vi "solar_voy_def Export (Packets).vi"(10 "HDR_ID_NAME ('HDR_ID')":string="HDR_ID", 11 "PACKETS":T1[](array[typedef]) {"last_time" format="%<%H:%M:%S%3u %m/%d/%y>T"}) -> (2 "Telemetry":string, 3 "Commands":string)   [LabVIEW 2018]
doc: "This exports packets to COSMOS definition strings."
uses:
  solar_voy_def_ctl ITEM TYPE.ctl
  type/solar_type Item Type.ctl
  solar_voy_def_ctl ITEM.ctl
  solar_voy_def_ctl PACKET_ID.ctl
  solar_voy_def_ctl PACKET.ctl
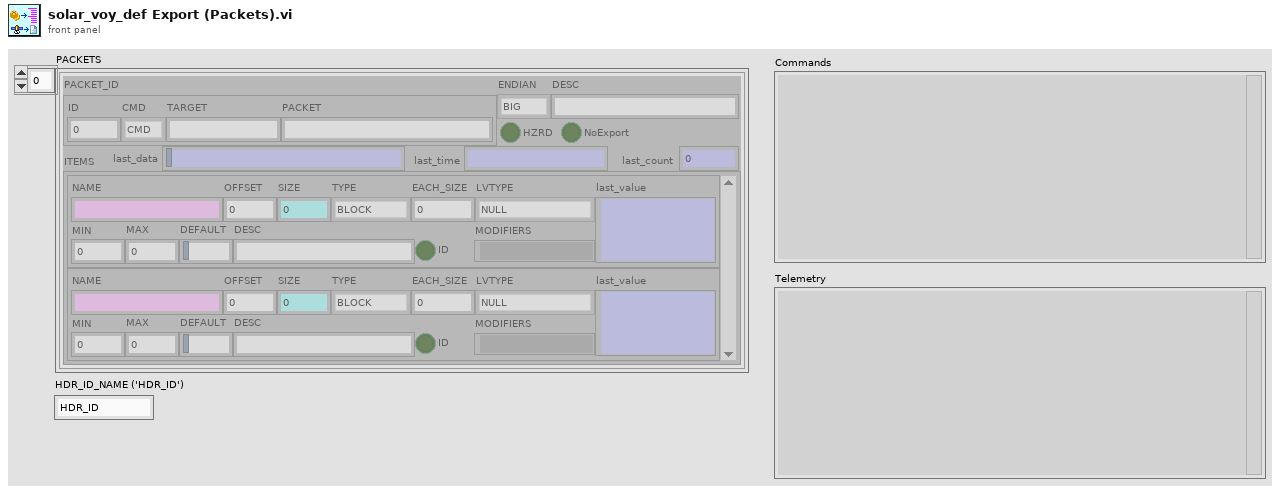
[diagram p1: front panel]
types:
  T1 = typedef "solar_voy_def_ctl PACKET.ctl" = cluster{"PACKET_ID":T2, "ENDIAN":enum8{"BIG", "LITTLE"}, "DESC":string, "HZRD":bool, "ITEMS":T3[], "NoExport":bool, "last_time":timestamp, "last_count":u32, "last_data":string}
  T2 = typedef "solar_voy_def_ctl PACKET_ID.ctl" = cluster{"ID":u16, "CMD":enum8{"CMD", "TLM"}, "TARGET":string, "PACKET":string}
  T3 = typedef "solar_voy_def_ctl ITEM.ctl" = cluster{"NAME":string, "OFFSET":i32, "SIZE":i32, "TYPE":T4, "EACH_SIZE":i32, "LVTYPE":T5, "MIN":dbl, "MAX":dbl, "DEFAULT":string, "DESC":string, "ID":bool, "MODIFIERS":variant, "last_value":variant}
  T4 = typedef "solar_voy_def_ctl ITEM TYPE.ctl" = enum8{"BLOCK", "INT", "UINT", "FLOAT", "STRING"}
  T5 = typedef "solar_type Item Type.ctl" = enum16{"NULL", "UNKNOWN", "CLUSTER", "I8", "I16", "I32", "I64", "U8", "U16", "U32", "U64", "U8_ENUM", "U16_ENUM", "U32_ENUM", "SGL", "DBL", "BOOLEAN", "STRING", "PATH", "VISA", "TAG", "TIME", "I8_1D", "I16_1D", "I32_1D", "I64_1D", "U8_1D", "U16_1D", "U32_1D", "U64_1D", "U8_ENUM_1D", "U16_ENUM_1D", "U32_ENUM_1D", "SGL_1D", "DBL_1D", "BOOLEAN_1D", "STRING_1D", "PATH_1D", "VISA_1D", "TAG_1D", "TIME_1D", "I8_2D", "I16_2D", "I32_2D", "I64_2D", "U8_2D", "U16_2D", "U32_2D", "U64_2D", "U8_ENUM_2D", "U16_ENUM_2D", "U32_ENUM_2D", "SGL_2D", "DBL_2D", "BOOLEAN_2D", "STRING_2D", "PATH_2D", "VISA_2D", "TAG_2D", "TIME_2D"}
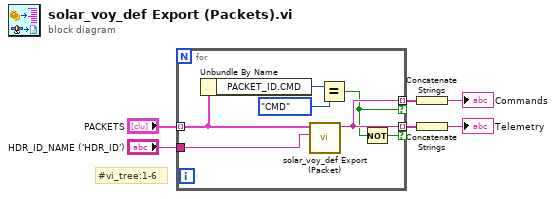
[diagram p0: block diagram]
diagram:
  # "#vi_tree:1-6"
  n1 = for {
    tunnel: "PACKETS" -> [w11] mode=indexing
    tunnel: [w13] -> w4 mode=indexing if=w8
    tunnel: [w13] -> w3 mode=indexing if=w12
    tunnel: "HDR_ID_NAME ('HDR_ID')" -> [w7]
    n2 = Unbundle By Name(w11) -> ("PACKET_ID.CMD"=w10:enum8{"CMD", "TLM"})
    n3 = call "solar_voy_def Export (Packet).vi"("HDR_ID_NAME ('HDR_ID')"=w7, "PACKET"=w11) -> ("PACKET Definition"=w13:string)  [unwired: 6 in, 3 out]
    n4 = Equal?(x=w10, y=enum8{"CMD", "TLM"}."CMD") -> (x = y?=w8:bool)
    n5 = Not(x=w8) -> (.not. x?=w12:bool)
  }
  n6 = Concatenate Strings(w4) -> (→"Commands":string)
  n7 = Concatenate Strings(w3) -> (→"Telemetry":string)
